vi "Read Step Data (DC Parallel L1N Manual Mode).vi"(0 "VISA resource name":refnum<visa-resource-name>, 5 "Step (1)":i32=1 min=1 max=9 format="%2_0f", 11 "error in (no error)":errorcluster) -> (4 "VISA resource name out":refnum<visa-resource-name>, 6 "Test Meter Data Output":T1 {"Voltage (V)" format="%.1f"; "RMS Current (A)" format="%.3f"; "Power (W)" format="%.1f"}, 15 "error out":errorcluster)   [LabVIEW 2016, in "APT 300XAC Series.lvlib"]
doc: "Reads the DC mode <B>Step data</B>. \n\nIn DC Mode the output data cluster has the following data.\n\n1. Memory\n2. Step\n3. Voltage (V)\n4. Current (A)\n5. Power (W)\n5. Status"
uses:
  APT 300XAC Series.lvlib
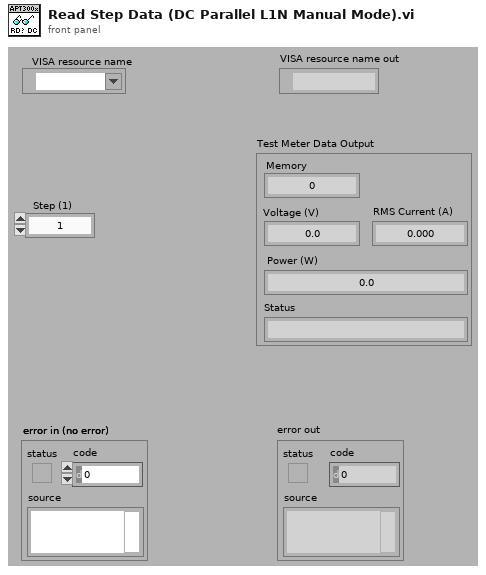
[diagram p1: front panel]
types:
  T1 = cluster{"Memory":dbl, "Voltage (V)":dbl, "RMS Current (A)":dbl, "Power (W)":dbl, "Status":string}
  T2 = cluster{"Memory":i32, "Volt":dbl, "Current":dbl, "Power":dbl, "Status":string}
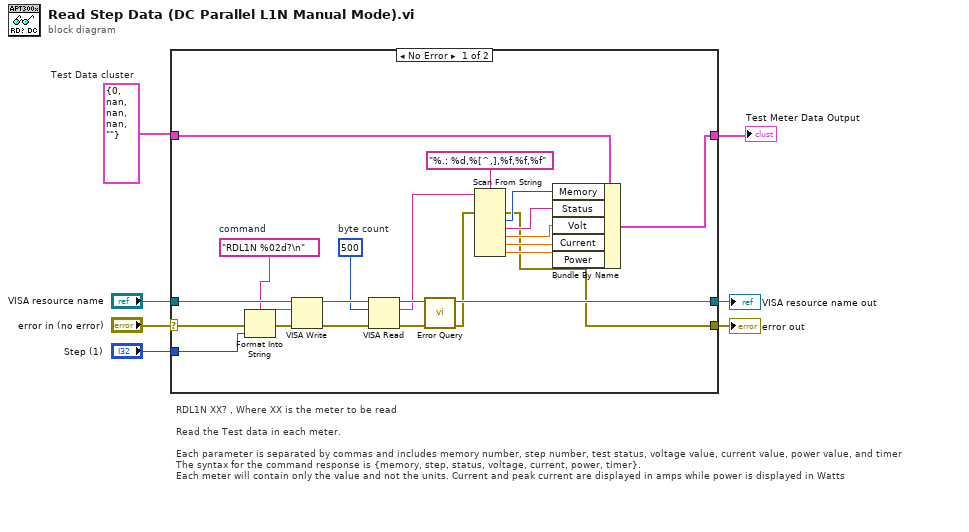
[diagram p0: block diagram]
diagram:
  w2 = T2 {"Memory"=0, "Volt"=nan, "Current"=nan, "Power"=nan, "Status"=""}  # Test Data cluster
  # "RDL1N XX? , Where XX is the meter to be read\n\nRead the Test data in each meter. \n\nEach parameter is separated by commas and includes memory number, step number, test status, voltage value, current value, power value, and timer\nThe syntax for the command response is {memory, step, status, voltage, current, power, timer}. \nEach meter will contain only the value and not the units. Current and peak current are displayed in amps while power is displayed in Watts"
  n1 = case shown="No Error" "error in (no error)" {
    selector: "error in (no error)" -> [w26 w32]
    tunnel: "VISA resource name" -> [w27 w33]
    tunnel: [w19 w33] -> w5
    tunnel: [w9 w32] -> w4
    tunnel: [w8 w31] -> w1
    tunnel: w2 -> [w12 w31]
    tunnel: "Step (1)" -> [w20 _]
    frame No Error {
      w22 = "RDL1N %02d?\n"  # command
      w28 = u32 500  # byte count
      n2 = Format Into String(format string=w22, error in=w26, w20) -> (resulting string=w21:string, error out=w23:errorcluster)  [unwired: 1 in]
      n3 = VISA Write(VISA resource name=w27, write buffer=w21, error in (no error)=w23) -> (VISA resource name out=w30:refnum<visa-resource-name>, error out=w29:errorcluster)  [unwired: 1 out]
      n4 = VISA Read(VISA resource name=w30, byte count=w28, error in (no error)=w29) -> (VISA resource name out=w25:refnum<visa-resource-name>, read buffer=w11:string, error out=w24:errorcluster)  [unwired: 1 out]
      n5 = call "Error Query.vi"("VISA resource name"=w25, "error in (no error)"=w24) -> ("VISA resource name out"=w19:refnum<visa-resource-name>, "error out"=w10:errorcluster)  [unwired: 10 in, 2 out]
      n6 = Scan From String(format string="%.; %d,%[^,],%f,%f,%f", input string=w11, error in=w10) -> (error out=w9:errorcluster, output 1=w17:i32, output 2=w16:string, output 3=w15:dbl, output 4=w14:dbl, output 5=w13:dbl)  [unwired: 6 in, 2 out]
      n7 = Bundle By Name(cluster=w12, "Memory"=w17, "Status"=w16, "Volt"=w15, "Current"=w14, "Power"=w13) -> (w8:T2)
    }
    frame Error {
    }
  }
  "VISA resource name out" <- w5
  "error out" <- w4
  "Test Meter Data Output" <- w1
